vi "Set.vi"(5 "Append Key? (F=Replace)":bool, 9 "Value [Scalar, Cluster, 1D_Clusters, 2D_String]":variant, 10 "Name":string, 11 "Variables in":map{string, string[]}(c390)) -> (2 "Replaced?":bool, 3 "Variables out":map{string, string[]}(c390))   [LabVIEW 2021, in "HttpServer.lvlib"]
uses:
  HttpServer.lvlib
  <vilib>/Utility/miscctls.llb/LVMapReplaceAction.ctl
  <vilib>/Utility/Data Type/NI_Data Type.lvlib
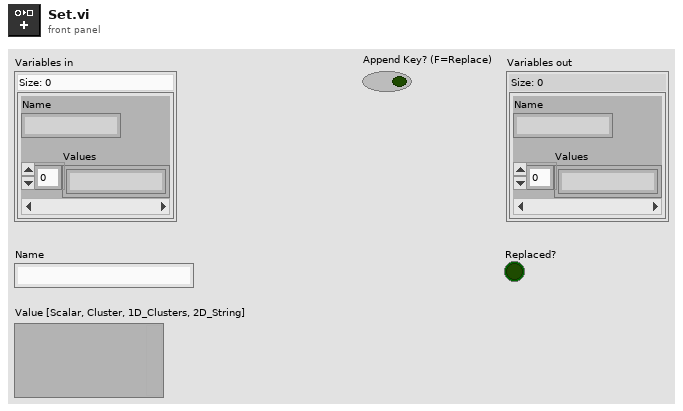
[diagram p1: front panel]
types:
  T1 = typedef "NI_Data Type.lvlib/Data Type.ctl" = enum8{"Invalid Type", "Void", "I8", "I16", "I32", "I64", "U8", "U16", "U32", "U64", "Single Float", "Double Float", "Extended Float", "Single Complex", "Double Complex", "Extended Complex", "Enum U8", "Enum U16", "Enum U32", "Enum U64", "Single Float With Unit", "Double Float With Unit", "Extended Float With Unit", "Single Complex with Unit", "Double Complex with Unit", "Extended Complex with Unit", "Boolean", "String", "Path", "Picture", "Tag", "Array", "Cluster", "Variant", "LV Variant", "Waveform", "Timestamp", "Digital Waveform", "Digital Data", "ExpressData", "Refnum", "External Data", "VI", "Poly VI", "LabVIEW Class Instance", "Fixed Point", "Set Collection", "Map Collection"}
  T2 = typedef "LVMapReplaceAction.ctl" = enum32{"Modify Entry only if found", "Add or Modify Entry", "Delete Entry"}
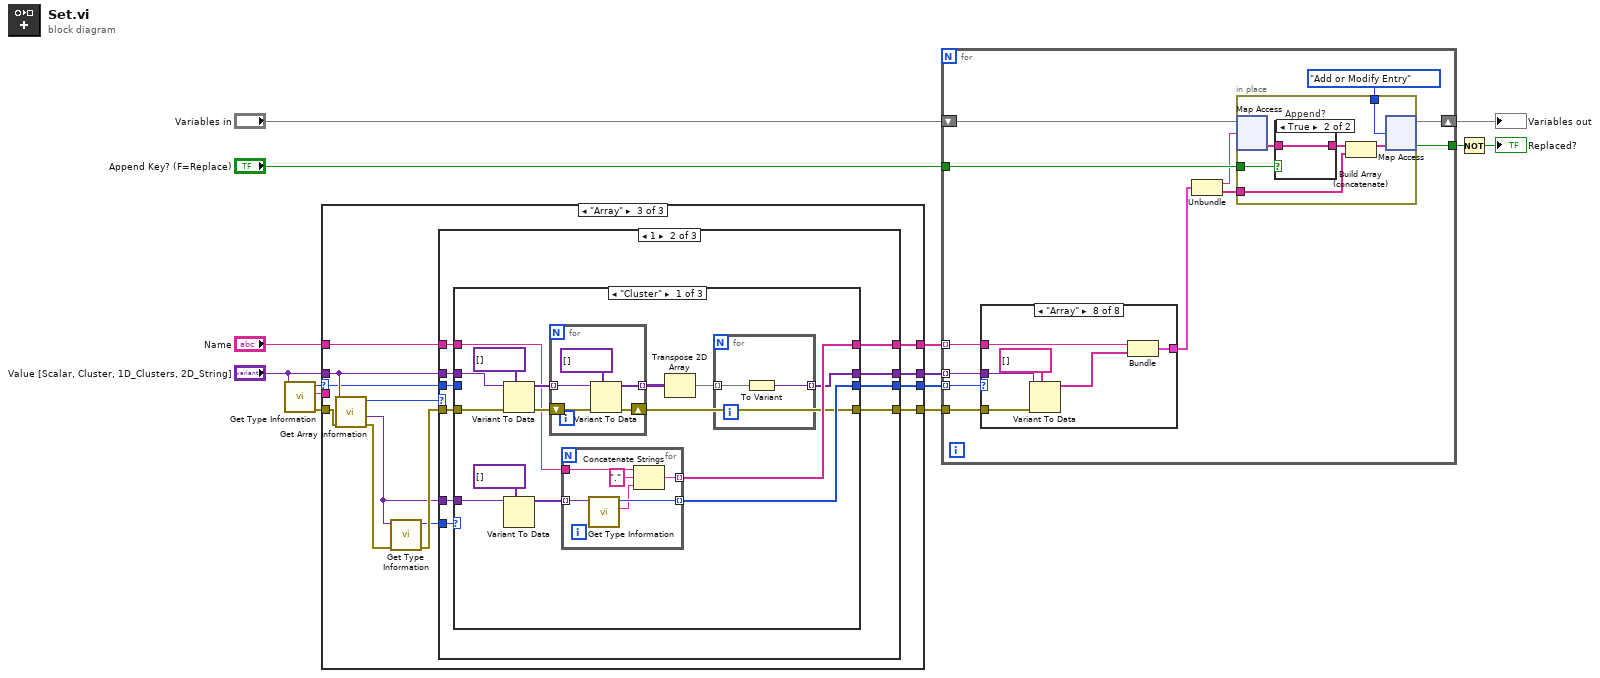
[diagram p0: block diagram]
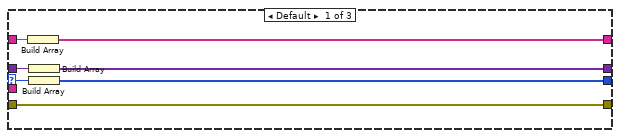
[diagram p2: hidden frame]
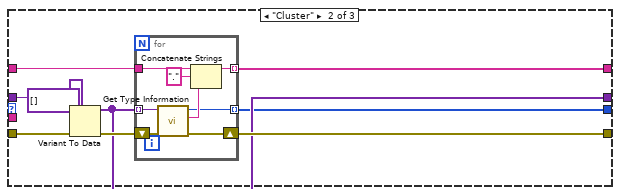
[diagram p3: hidden frame]
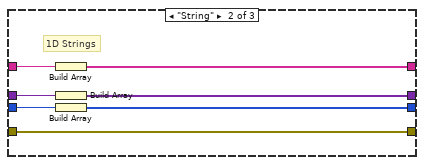
[diagram p5: hidden frame]
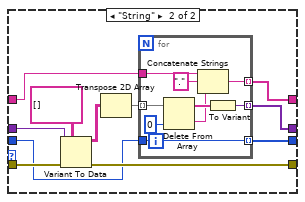
[diagram p8: hidden frame]
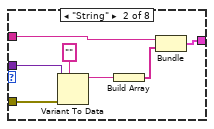
[diagram p11: hidden frame]
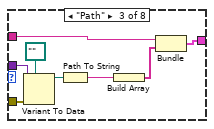
[diagram p12: hidden frame]
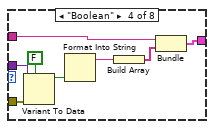
[diagram p13: hidden frame]
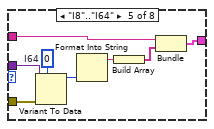
[diagram p14: hidden frame]
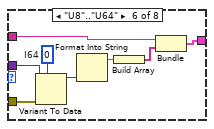
[diagram p15: hidden frame]
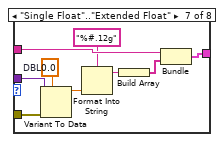
[diagram p16: hidden frame]
diagram:
  n1 = call <vilib>:"Get Type Information.vi"("variant"="Value [Scalar, Cluster, 1D_Clusters, 2D_String]") -> ("error out"=w9:errorcluster, "name"=w2:string, "type"=w10:T1)  [unwired: 6 in, 2 out]
  n2 = case shown="\"Array\"" w10 {
    selector: w10 -> [w16 _ w41]
    tunnel: "Value [Scalar, Cluster, 1D_Clusters, 2D_String]" -> [w21 w28 w48]
    tunnel: w9 -> [w19 w29 w49]
    tunnel: [w19 w26 w51] -> w6
    tunnel: [w20 w23 w50] -> w7
    tunnel: "Name" -> [w17 w25 w42]
    tunnel: [w18 w24 w43] -> w8
    tunnel: w2 -> [_ _ _]
    tunnel: [w15 w22 w40] -> w1
    frame Default {
      n3 = Build Array(w17) -> (w18:string[])
      n4 = Build Array(w21) -> (w20:variant[])
      n5 = Build Array(w16) -> (w15:T1[])
    }
    frame "Cluster" {
      n6 = Variant To Data(error in=w29, type=variant[] [], Variant=w28) -> (data=w23:variant[], error out=w27:errorcluster)
      n7 = for {
        tunnel: w23 -> [w37] mode=indexing
        shift-right: [w36] -> w26
        shift-left: w27 -> [w38]
        tunnel: w25 -> [w33]
        tunnel: [w34] -> w24 mode=indexing
        tunnel: [w31] -> w22 mode=indexing
        n8 = call <vilib>:"Get Type Information.vi"("error in (no error)"=w38, "variant"=w37) -> ("error out"=w36:errorcluster, "name"=w35:string, "type"=w31:T1)  [unwired: 5 in, 2 out]
        n9 = Concatenate Strings(w33, "." ("string"), w35) -> (w34:string)
      }
    }
    frame "Array" {
      n10 = call <vilib>:"Get Array Information.vi"("error in (no error)"=w49, "variant"=w48) -> ("error out"=w47:errorcluster, "array element data type"=w39:variant, "number of dimensions"=w45:i32)  [unwired: 6 in, 1 out]
      n11 = call <vilib>:"Get Type Information.vi"("error in (no error)"=w47, "variant"=w39) -> ("error out"=w46:errorcluster, "type"=w44:T1)  [unwired: 5 in, 3 out]
      n12 = case shown="1" w45 {
        tunnel: [w52 w62 w106] -> w51
        tunnel: [_ w61 w103] -> w50
        tunnel: w48 -> [_ w60 w105]
        tunnel: w46 -> [w52 w59 w107]
        tunnel: w44 -> [_ w58 w104]
        tunnel: [_ w56 w102] -> w43
        tunnel: w42 -> [_ w57 w101]
        tunnel: w41 -> [_ w55 w99]
        tunnel: [_ w54 w100] -> w40
        tunnel: w39 -> [_ w53 _]
        frame Default {
          # "Not\nSupported"
        }
        frame 1 {
          n13 = case shown="\"Cluster\"" w58 {
            tunnel: [w65 w97 w98] -> w62
            tunnel: [w63 w95 _] -> w61
            tunnel: w60 -> [w75 w96 _]
            tunnel: w59 -> [w76 w97 w98]
            tunnel: w57 -> [w68 w94 _]
            tunnel: [w67 w93 _] -> w56
            tunnel: w55 -> [_ w92 _]
            tunnel: [w66 w91 _] -> w54
            tunnel: w53 -> [w71 _ _]
            frame "Cluster" {
              n14 = Variant To Data(error in=w76, type=variant[] [], Variant=w75) -> (data=w73:variant[], error out=w74:errorcluster)
              n15 = Variant To Data(type=variant[] [], Variant=w71) -> (data=w69:variant[])  [unwired: 1 in, 1 out]
              n16 = for {
                shift-right: [w87] -> w65
                shift-left: w74 -> [w90]
                tunnel: w73 -> [w88] mode=indexing
                tunnel: [w86] -> w70 mode=indexing
                n17 = Variant To Data(error in=w90, type=variant[] [], Variant=w88) -> (data=w86:variant[], error out=w87:errorcluster)
              }
              n18 = for {
                tunnel: w69 -> [w80] mode=indexing
                tunnel: [w81] -> w67 mode=indexing
                tunnel: [w85] -> w66 mode=indexing
                tunnel: w68 -> [w83]
                n19 = call <vilib>:"Get Type Information.vi"("variant"=w80) -> ("name"=w82:string, "type"=w85:T1)  [unwired: 6 in, 3 out]
                n20 = Concatenate Strings(w83, "." ("string"), w82) -> (w81:string)
              }
              n21 = Transpose 2D Array(2D array=w70) -> (transposed array=w64:variant[][])
              n22 = for {
                tunnel: w64 -> [w79] mode=indexing
                tunnel: [w78] -> w63 mode=indexing
                n23 = To Variant(anything=w79) -> (Variant=w78:variant)
              }
            }
            frame "String" {
              # "1D Strings"
              n24 = Build Array(w94) -> (w93:string[])
              n25 = Build Array(w96) -> (w95:variant[])
              n26 = Build Array(w92) -> (w91:T1[])
            }
            frame Default {
              # "Not\nSupported"
            }
          }
        }
        frame 2 {
          n27 = case shown="Default" w104 {
            tunnel: w107 -> [w108 w119]
            tunnel: [w108 w118] -> w106
            tunnel: w105 -> [_ w117]
            tunnel: [_ w113] -> w103
            tunnel: [_ w112] -> w102
            tunnel: w101 -> [_ w111]
            tunnel: [_ w109] -> w100
            tunnel: w99 -> [_ w110]
            frame Default {
            }
            frame "String" {
              n28 = Variant To Data(error in=w119, type=string[][] [], Variant=w117) -> (data=w115:string[][], error out=w118:errorcluster)
              n29 = Transpose 2D Array(2D array=w115) -> (transposed array=w114:string[][])
              n30 = for {
                tunnel: w114 -> [w128] mode=indexing
                tunnel: [w125] -> w113 mode=indexing
                tunnel: [w123] -> w112 mode=indexing
                tunnel: w111 -> [w121]
                tunnel: [w120] -> w109 mode=indexing
                tunnel: w110 -> [w120]
                n31 = Delete From Array(array=w128, index=0) -> (deleted portion=w124:string, array with subset deleted=w126:string[])  [unwired: 1 in]
                n32 = Concatenate Strings(w121, "." ("string"), w124) -> (w123:string)
                n33 = To Variant(anything=w126) -> (Variant=w125:variant)
              }
            }
          }
        }
      }
    }
  }
  n34 = for {
    tunnel: w7 -> [w140] mode=indexing
    tunnel: w8 -> [w133] mode=indexing
    tunnel: w6 -> [w134]
    shift-right: [w137] -> w3
    shift-left: "Variables in" -> [w138]
    tunnel: [w129] -> w13
    tunnel: w1 -> [w135] mode=indexing
    tunnel: "Append Key? (F=Replace)" -> [w136]
    n35 = case shown="\"Array\"" w135 {
      tunnel: w134 -> [_ w154 w162 w170 w178 w186 w195 w201]
      tunnel: w140 -> [_ w152 w161 w169 w177 w185 w194 w199]
      tunnel: w133 -> [_ w149 w158 w167 w175 w183 w192 w198]
      tunnel: [_ w148 w157 w166 w174 w182 w191 w197] -> w139
      frame Default {
      }
      frame "String" {
        n36 = Variant To Data(error in=w154, type="", Variant=w152) -> (data=w151:string)  [unwired: 1 out]
        n37 = Build Array(w151) -> (w150:string[])
        n38 = Bundle("Name"=w149, w150) -> (w148:cluster{"Name":string, string[]})  [unwired: 1 in]
      }
      frame "Path" {
        n39 = Variant To Data(error in=w162, type=path "", Variant=w161) -> (data=w160:path)  [unwired: 1 out]
        n40 = Path To String(path=w160) -> (string=w155:string)
        n41 = Build Array(w155) -> (w159:string[])
        n42 = Bundle("Name"=w158, w159) -> (w157:cluster{"Name":string, string[]})  [unwired: 1 in]
      }
      frame "Boolean" {
        n43 = Variant To Data(error in=w170, type=FALSE, Variant=w169) -> (data=w164:bool)  [unwired: 1 out]
        n44 = Format Into String(w164) -> (resulting string=w163:string)  [unwired: 3 in, 1 out]
        n45 = Build Array(w163) -> (w168:string[])
        n46 = Bundle("Name"=w167, w168) -> (w166:cluster{"Name":string, string[]})  [unwired: 1 in]
      }
      frame "I8".."I64" {
        w173 = i64 0  # I64
        n47 = Variant To Data(error in=w178, type=w173, Variant=w177) -> (data=w172:i64)  [unwired: 1 out]
        n48 = Format Into String(w172) -> (resulting string=w171:string)  [unwired: 3 in, 1 out]
        n49 = Build Array(w171) -> (w176:string[])
        n50 = Bundle("Name"=w175, w176) -> (w174:cluster{"Name":string, string[]})  [unwired: 1 in]
      }
      frame "U8".."U64" {
        w181 = i64 0  # I64
        n51 = Variant To Data(error in=w186, type=w181, Variant=w185) -> (data=w180:i64)  [unwired: 1 out]
        n52 = Format Into String(w180) -> (resulting string=w179:string)  [unwired: 3 in, 1 out]
        n53 = Build Array(w179) -> (w184:string[])
        n54 = Bundle("Name"=w183, w184) -> (w182:cluster{"Name":string, string[]})  [unwired: 1 in]
      }
      frame "Single Float".."Extended Float" {
        w190 = 0.0  # DBL
        n55 = Variant To Data(error in=w195, type=w190, Variant=w194) -> (data=w189:dbl)  [unwired: 1 out]
        n56 = Format Into String(format string="%#.12g", w189) -> (resulting string=w188:string)  [unwired: 2 in, 1 out]
        n57 = Build Array(w188) -> (w193:string[])
        n58 = Bundle("Name"=w192, w193) -> (w191:cluster{"Name":string, string[]})  [unwired: 1 in]
      }
      frame "Array" {
        n59 = Variant To Data(error in=w201, type=string[] [], Variant=w199) -> (data=w196:string[])  [unwired: 1 out]
        n60 = Bundle("Name"=w198, w196) -> (w197:cluster{"Name":string, string[]})  [unwired: 1 in]
      }
    }
    n61 = Unbundle(w139) -> ("Name"=w132:string, w131:string[])
    n62 = in-place {
      in-place-border: w131 -> [w144]
      in-place-border: LVMapReplaceAction."Add or Modify Entry" ("action") -> [w146]
      in-place-border: w136 -> [w141]
      n63 = in-place-map #1(w138, w132) -> (w143:string[])  [unwired: 1 in, 1 out]
      n64 = case "Append?" shown="True" w141 {
        tunnel: [_ w147] -> w142
        tunnel: w143 -> [_ w147]
        frame False {
        }
        frame True {
        }
      }
      n65 = Build Array (concatenate)(w142, w144) -> (w145:string[])
      n66 = in-place-map #1(w145, w146) -> (w137:map{string, string[]}, w129:bool)  [unwired: 1 out]
    }
  }
  "Variables out" <- w3
  n67 = Not(x=w13) -> (.not. x?=→"Replaced?":bool)
